vi "CreatePreprocFile.vi"(8 "error in (no error)":errorcluster, 10 "Python Instruction":string, 11 "Python in":refnum<class "Python.lvclass">) -> (0 "error out":errorcluster, 3 "Python out":refnum<class "Python.lvclass">)   [LabVIEW 2020, in "Python.lvclass"]
uses:
  Python.lvclass
  Python.lvclass/Python.ctl
panel:
  out "appended path":path
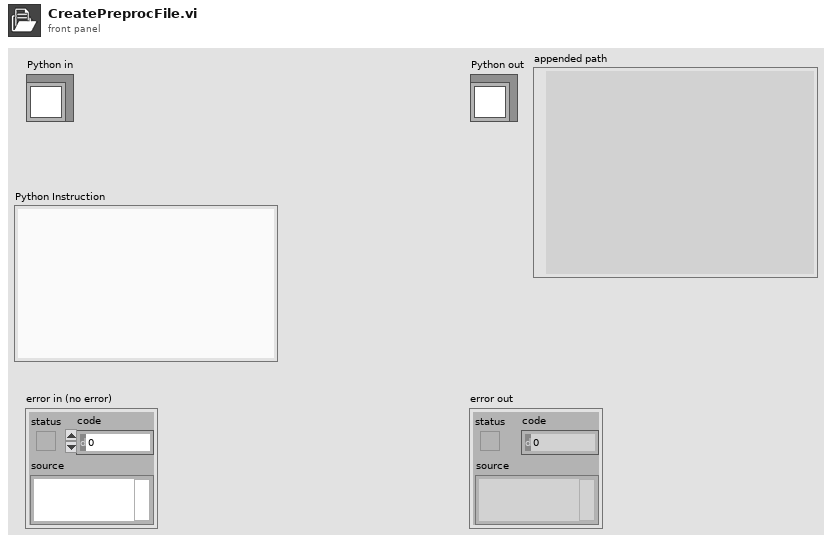
[diagram p1: front panel]
types:
  T1 = enum16{"open", "replace", "create", "open or create", "replace or create", "replace or create with confirmation"}
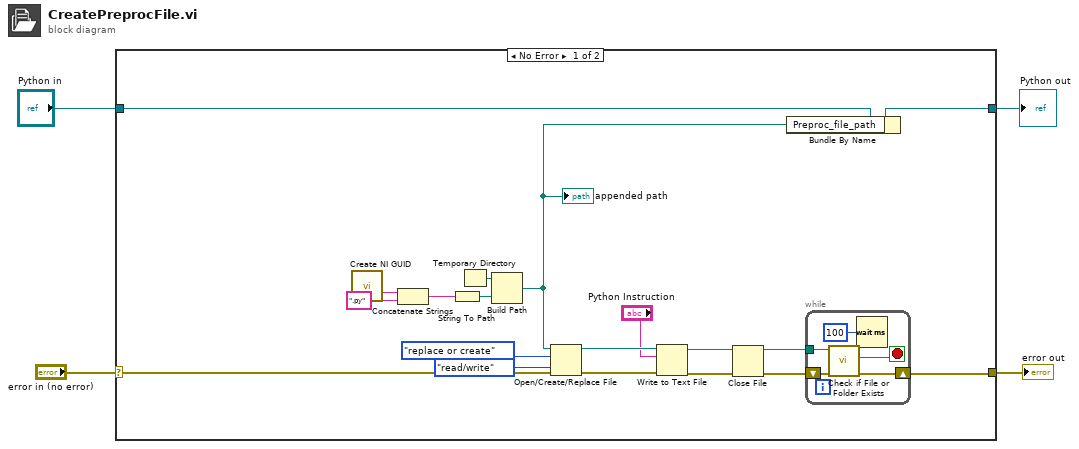
[diagram p0: block diagram]
diagram:
  n1 = case shown="No Error" "error in (no error)" {
    selector: "error in (no error)" -> [w21 w30]
    tunnel: [w8 w30] -> w3
    tunnel: [w22 w29] -> w1
    tunnel: "Python in" -> [w23 w29]
    frame No Error {
      n2 = call <vilib>:"Create NI GUID.vi"() -> ("NI GUID"=w5:string)
      n3 = Concatenate Strings(w5, ".py" ("string")) -> (w6:string)
      n4 = String To Path(string=w6) -> (path=w13:path)
      n5 = Temporary Directory() -> (w11:path)
      n6 = Build Path(base path=w11, name or relative path=w13) -> (appended path=w9:path)
      "appended path" <- w9
      n7 = Open/Create/Replace File(file path (use dialog)=w9, error in=w21, operation (0:open)=T1."replace or create", access (0:read/write)=enum16{"read/write", "read-only", "write-only"}."read/write") -> (refnum out=w17:refnum<file>, error out=w20:errorcluster)  [unwired: 2 in, 1 out]
      n8 = Write to Text File(file (use dialog)=w17, text="Python Instruction", error in=w20) -> (refnum out=w18:refnum<file>, error out=w19:errorcluster)  [unwired: 1 in, 1 out]
      n9 = Close File(refnum=w18, error in=w19) -> (path=w7:path, error out=w10:errorcluster)
      n10 = Bundle By Name(cluster=w23, "Preproc_file_path"=w9) -> (w22:refnum<class "Python.lvclass">)
      n11 = while {
        tunnel: w7 -> [w27]
        shift-right: [w26] -> w8
        shift-left: w10 -> [w28]
        stop <- w25 stop-if-true
        n12 = call <vilib>:"Check if File or Folder Exists.vi"("error in (no error)"=w28, "path"=w27) -> ("error out"=w26:errorcluster, "file or folder exists?"=w25:bool)  [unwired: 7 in, 1 out]
        n13 = Wait (ms)(milliseconds to wait=u32 100) -> ()  [unwired: 1 out]
      }
    }
    frame Error {
    }
  }
  "error out" <- w3
  "Python out" <- w1
